vi "Interlocks.vi"(7 "Action":enum16{"Initialize", "Update"}(ring), 8 "error in (no error)":errorcluster, 9 "Override? (F)":bool, 10 "Variables":refnum<vi>[](array[refnum]), 11 "Interlocks (.ini)":path) -> (0 "error out":errorcluster)   [LabVIEW 2022 SP3, in "Interlocks.lvlib"]
uses:
  Interlocks.lvlib
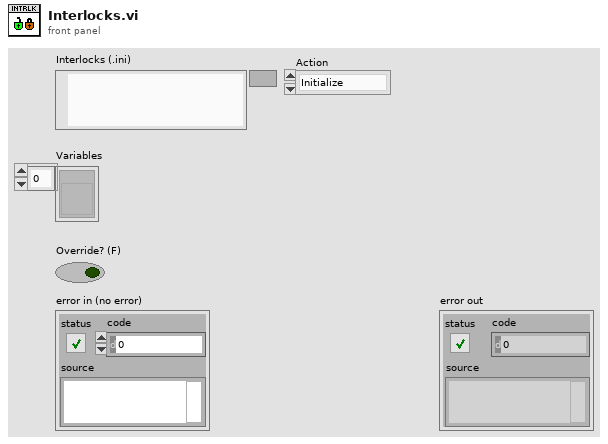
[diagram p1: front panel]
types:
  T1 = enum8{"Enabled", "Disabled", "Disabled and Grayed Out"}
  T2 = enum8{"Enabled", "Disabled", "Disabled and Grayed Out"}[]
  T3 = typedef "Interlocks.lvlib/Interlock.ctl" = cluster{"Types":T4[], "Values":dbl[]}
  T4 = typedef "Interlocks.lvlib/Token Type.ctl" = enum8{"INVALID", "NOT", "AND", "OR", "EE", "NE", "LT", "GT", "LTE", "GTE", "PLUS", "MINUS", "MULTIPLY", "DIVIDE", "MODULUS", "LPAREN", "RPAREN", "LITERAL", "IDENTIFIER", "DEFINITION"}
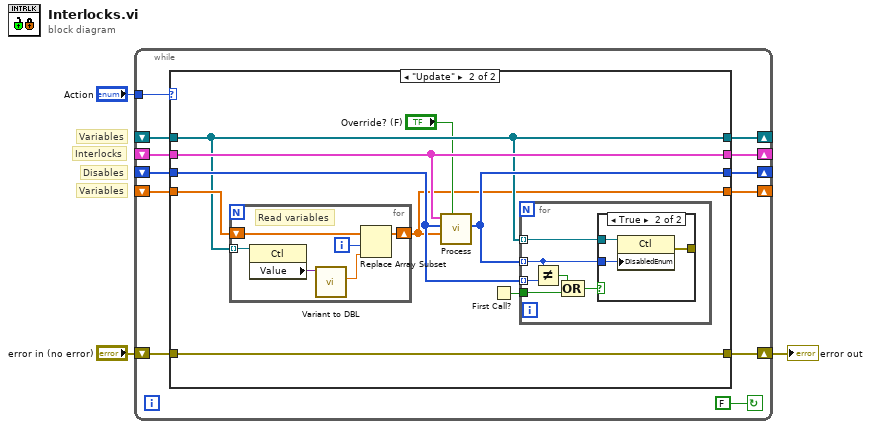
[diagram p0: block diagram]
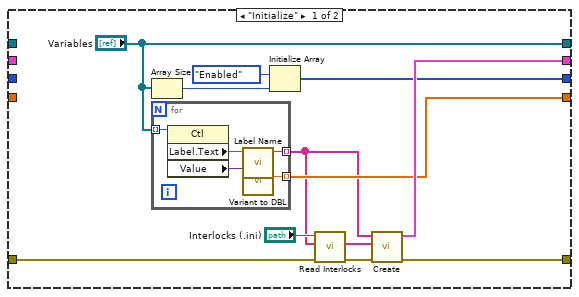
[diagram p2: hidden frame]
diagram:
  # "Variables"
  # "Disables"
  # "Interlocks"
  # "Variables"
  n1 = while {
    shift-right: [w15] -> w3
    shift-left: "error in (no error)" -> [w14]
    tunnel: "Action" -> [w12]
    shift-right: [w11] -> _
    shift-left: _ -> [w10]
    shift-right: [w8] -> _
    shift-left: _ -> [w9]
    shift-right: [w7] -> _
    shift-left: _ -> [w6]
    shift-right: [w5] -> _
    shift-left: _ -> [w4]
    stop <- FALSE continue-if-true
    n2 = case shown="\"Update\"" w12 {
      tunnel: [w24 w41] -> w15
      tunnel: w14 -> [w19 w41]
      tunnel: ["Variables" w35] -> w11
      tunnel: w10 -> [_ w35]
      tunnel: w9 -> [_ w39]
      tunnel: [w27 w39] -> w8
      tunnel: [w26 w36] -> w7
      tunnel: w6 -> [_ w37]
      tunnel: [w23 w33] -> w5
      tunnel: w4 -> [_ w40]
      frame "Initialize" {
        n3 = Array Size(array="Variables") -> (size(s)=w25:i32)
        n4 = for {
          tunnel: "Variables" -> [w32] mode=indexing
          tunnel: [w30] -> w16 mode=indexing
          tunnel: [w28] -> w23 mode=indexing
          n5 = property class="Ctl"(reference=w32) -> ("Label.Text"=w31:string, "Value"=w29:variant)  [unwired: 1 in, 2 out]
          n6 = call "Label Name.vi"("Label Text"=w31) -> ("Variable Name"=w30:string)  [unwired: 10 in]
          n7 = call "Variant to DBL.vi"("Variant"=w29) -> ("Value as DBL"=w28:dbl)  [unwired: 9 in, 1 out]
        }
        n8 = Initialize Array(T1."Enabled" ("Disabled"), w25) -> (w26:T2)
        n9 = call "Read Interlocks.vi"("error in (no error)"=w19, "Variable Names"=w16, "Interlocks (.ini)"="Interlocks (.ini)") -> ("error out"=w20:errorcluster, "Variable Interlocks"=w17:string[])  [unwired: 6 in, 1 out]
        n10 = call "Create.vi"("error in (no error)"=w20, "Variable Interlocks"=w17, "Variable Names"=w16) -> ("error out"=w24:errorcluster, "Interlocks"=w27:T3[])  [unwired: 7 in]
      }
      frame "Update" {
        n11 = for {
          tunnel: w35 -> [w47] mode=indexing
          shift-right: [w42] -> w33
          shift-left: w40 -> [w44]
          i -> [w43]
          # "Read variables"
          n12 = property class="Ctl"(reference=w47) -> ("Value"=w46:variant)  [unwired: 1 in, 2 out]
          n13 = call "Variant to DBL.vi"("Variant"=w46) -> ("Value as DBL"=w45:dbl)  [unwired: 9 in, 1 out]
          n14 = Replace Array Subset(array=w44, new element=w45, index=w43) -> (w42:dbl[])
        }
        n15 = call "Process.vi"("Override? (F)"="Override? (F)", "Values in"=w33, "Disabled in"=w37, "Interlocks"=w39) -> ("Disabled out"=w36:T2)  [unwired: 7 in]
        n16 = First Call?() -> (First Call?: T/F=w38:bool)
        n17 = for {
          tunnel: w35 -> [w48] mode=indexing
          tunnel: w36 -> [w53] mode=indexing
          tunnel: w37 -> [w51] mode=indexing
          tunnel: w38 -> [w49]
          n18 = Not Equal?(x=w53, y=w51) -> (x != y?=w52:bool)
          n19 = Compound Arithmetic op=OR(w52, w49) -> (w50:bool)
          n20 = case shown="True" w50 {
            tunnel: w53 -> [_ w54]
            tunnel: w48 -> [_ w56]
            tunnel: [_ w55] -> _
            frame False {
            }
            frame True {
              n21 = property class="Ctl"(reference=w56, "DisabledEnum"=w54) -> (error out=w55:errorcluster)  [unwired: 1 in, 1 out]
            }
          }
        }
      }
    }
  }
  "error out" <- w3
